vi "ATCcont.vi"() -> ()   [LabVIEW 2014]
doc: "ATC app"
panel:
  in  "정지":bool
  in  "정보1":bool
  in  "도움말":bool
  in  "?":bool
  in  "?":bool
  in  "탭":T1(tab)
  in  "메모":string="필요한 메모를 할수 있습니다. "
  in  "SID&RadarVector. 2":string="SID&RadarVector. "
  in  "인사말":string="인사말"
  in  "CD관제기관":string="관제기관"
  in  "콜사인":string="콜사인\n콜사인\n콜사인"
  in  "도착공항":string="도착공항"
  in  "SID&RadarVector":string="SID&RadarVector"
  in  "비행고도":string="비행고도"
  in  "인사말2":string="인사말"
  in  "콜사인2":string="콜사인"
  in  "콜사인3":string="콜사인"
  in  "콜사인4":string="콜사인"
  in  "콜사인5":string="콜사인"
  in  "콜사인6":string="콜사인"
  in  "도착공항2":string="도착공항"
  in  "제한고도":string="제한고도"
  in  "비행고도2":string="비행고도"
  in  "D접속주파수":string="접속주파수"
  in  "스콱번호":string="스콱번호"
  in  "도착공항3":string="도착공항"
  in  "SID&RadarVector. 3":string="SID&RadarVector. "
  in  "제한고도2":string="제한고도"
  in  "비행고도3":string="비행고도"
  in  "D접속주파수2":string="접속주파수"
  in  "스콱번호2":string="스쾃번호"
  in  "콜사인7":string="콜사인"
  in  "콜사인8":string="콜사인"
  in  "G관제기관":string="관제기관"
  in  "G접속주파수2":string="접속주파수"
  in  "G관제기관2":string="관제기관"
  in  "G접속주파수":string="접속주파수"
  in  "콜사인9":string="콜사인"
  in  "유도로 2":string="유도로"
  in  "유도로":string="유도로"
  in  "방향 2":string="방향"
  in  "방향":string="방향"
  in  "메모2":string="필요한 메모를 할수 있습니다. "
  in  "T관제기관2":string="관제기관"
  in  "콜사인24":string="콜사인"
  in  "T접속주파수2":string="접속주파수"
  in  "T접속주파수":string="접속주파수"
  in  "T관제기관":string="관제기관"
  in  "콜사인23":string="콜사인"
  in  "활주로9":string="활주로"
  in  "G관제기관4":string="관제기관"
  in  "콜사인22":string="콜사인"
  in  "콜사인21":string="콜사인"
  in  "콜사인20":string="콜사인"
  in  "콜사인19":string="콜사인"
  in  "활주로8":string="활주로"
  in  "활주로7":string="활주로"
  in  "콜사인17":string="콜사인"
  in  "활주로6":string="활주로"
  in  "콜사인18":string="콜사인"
  in  "활주로5":string="활주로"
  in  "콜사인16":string="콜사인"
  in  "활주로4":string="활주로"
  in  "콜사인15":string="콜사인"
  in  "활주로3":string="활주로"
  in  "콜사인14":string="콜사인"
  in  "콜사인13":string="콜사인"
  in  "현재기압2":string="현재기압"
  in  "출발공항":string="출발공항"
  in  "활주로2":string="활주로"
  in  "현재기압":string="현재기압"
  in  "출발공항2":string="출발공항"
  in  "활주로1":string="활주로"
  in  "콜사인12":string="콜사인"
  in  "콜사인11":string="콜사인"
  in  "G관제기관3":string="관제기관"
  in  "인사3":string="인사"
  in  "콜사인34 2":string="콜사인"
  in  "D관제기관2":string="관제기관"
  in  "D관제기관":string="관제기관"
  in  "T관제기관3":string="관제기관"
  in  "메모3":string="필요한 메모를 할수 있습니다. "
  in  "인사4":string="인사"
  in  "콜사인25":string="콜사인"
  in  "활주로10":string="활주로"
  in  "콜사인26":string="콜사인"
  in  "바람방향":string="바람방향"
  in  "풍속":string="풍속"
  in  "콜사인28":string="콜사인"
  in  "활주로13":string="활주로"
  in  "콜사인29":string="콜사인"
  in  "활주로12":string="활주로"
  in  "콜사인30":string="콜사인"
  in  "활주로14":string="활주로"
  in  "콜사인31":string="콜사인"
  in  "활주로15":string="활주로"
  in  "T관제기관4":string="관제기관"
  in  "콜사인32":string="콜사인"
  in  "현재고도":string="현재고도"
  in  "허가고도":string="허가고도"
  in  "콜사인33":string="콜사인"
  in  "접속주파수":string="접속주파수"
  in  "콜사인34":string="콜사인"
  in  "접속주파수2":string="접속주파수"
  in  "순항고도or이니셜고도":string="순항고도or이니셜고도"
  in  "D관제기관5":string="관제기관"
  in  "메모 4":string="필요한 메모를 할수 있습니다. "
  in  "인사5":string="인사"
  in  "D관제기관3":string="관제기관"
  in  "콜사인35":string="콜사인"
  in  "현재고도A":string="현재고도"
  in  "콜사인36":string="콜사인"
  in  "D관제기관4":string="관제기관"
  in  "허가고도4":string="허가고도"
  in  "허가고도5":string="허가고도"
  in  "콜사인37":string="콜사인"
  in  "콜사인38":string="콜사인"
  in  "허가고도6":string="허가고도"
  in  "허가고도7":string="허가고도"
  in  "콜사인39":string="콜사인"
  in  "콜사인40":string="콜사인"
  in  "C관제기관":string="관제기관"
  in  "A접속주파수":string="접속주파수"
  in  "C관제기관2":string="관제기관"
  in  "A접속주파수2":string="접속주파수"
  in  "콜사인41":string="콜사인"
  in  "콜사인38 2":string="콜사인"
  in  "D관제기관6":string="관제기관"
  in  "허가고도6 2":string="허가고도"
  in  "허가고도6 3":string="허가고도"
  in  "콜사인39 2":string="콜사인"
  in  "메모5":string="필요한 메모를 할수 있습니다. "
  in  "인사말 2":string="인사말"
  in  "허가고도 2":string="허가고도"
  in  "지점":string="지점"
  in  "허가고도7 2":string="허가고도"
  in  "콜사인38 3":string="콜사인"
  in  "콜사인39 3":string="콜사인"
  in  "허가고도7 3":string="허가고도"
  in  "지점 2":string="지점"
  in  "메모6":string="필요한 메모를 할수 있습니다. "
  in  "A관제기관3":string="관제기관"
  in  "콜사인46":string="콜사인"
  in  "날시정보":string="날시정보"
  in  "고도":string="고도"
  in  "콜사인47":string="콜사인"
  in  "A관제기관4":string="관제기관"
  in  "L활주로":string="활주로"
  in  "도착공항4":string="도착공항"
  in  "현재기압":string="현재기압"
  in  "콜사인48":string="콜사인"
  in  "A관제기관5":string="관제기관"
  in  "L활주로":string="활주로"
  in  "도착공항5":string="도착공항"
  in  "현재기압":string="현재기압"
  in  "콜사인49":string="콜사인"
  in  "고도":string="고도"
  in  "콜사인50":string="콜사인"
  in  "고도":string="고도"
  in  "콜사인51":string="콜사인"
  in  "고도":string="고도"
  in  "고도":string="고도"
  in  "콜사인52":string="콜사인"
  in  "콜사인53":string="콜사인"
  in  "A관제기관":string="관제기관"
  in  "풍속":string="풍속"
  in  "바람방향":string="바람방향"
  in  "L활주로3":string="활주로"
  in  "콜사인54":string="콜사인"
  in  "L활주로":string="활주로"
  in  "콜사인55":string="콜사인"
  in  "A관제기관2":string="관제기관"
  in  "L활주로":string="활주로"
  in  "ILS":string="주파수(ils)"
  in  "콜사인56":string="콜사인"
  in  "L활주로6":string="활주로"
  in  "ILS2":string="주파수(ils)"
  in  "콜사인57":string="콜사인"
  in  "T관제기관":string="관제기관"
  in  "T접속주파수":string="접속주파수"
  in  "콜사인58":string="콜사인"
  in  "콜사인59":string="콜사인"
  in  "관제기관":string="관제기관"
  in  "T접속주파수":string="접속주파수"
  in  "메모7":string="필요한 메모를 할수 있습니다. "
  in  "바람방향":string="바람방향"
  in  "관제기관":string="관제기관"
  in  "콜사인60":string="콜사인"
  in  "L활주로7":string="활주로"
  in  "콜사인61":string="콜사인"
  in  "풍속":string="풍속"
  in  "콜사인62":string="콜사인"
  in  "L활주로":string="활주로"
  in  "L활주로":string="활주로"
  in  "관제기관":string="관제기관"
  in  "콜사인63":string="콜사인"
  in  "관제기관3":string="관제기관"
  in  "콜사인64":string="콜사인"
  in  "L활주로":string="활주로"
  in  "G관제기관":string="관제기관"
  in  "G접속주파수":string="접속주파수"
  in  "콜사인65":string="콜사인"
  in  "관제기관":string="관제기관"
  in  "G접속주파수":string="접속주파수"
  in  "콜사인70":string="콜사인"
  in  "C활주로3":string="활주로"
  in  "C활주로2":string="활주로"
  in  "관제기관3 2":string="관제기관"
  in  "C활주로":string="활주로"
  in  "콜사인69":string="콜사인"
  in  "관제기관2":string="관제기관"
  in  "메모8":string="필요한 메모를 할수 있습니다. "
  in  "관제기관":string="관제기관"
  in  "콜사인66":string="콜사인"
  in  "콜사인67":string="콜사인"
  in  "게이트번호":string="게이트번호"
  in  "THEN":string="then"
  in  "콜사인68":string="콜사인"
  in  "게이트번호2":string="게이트번호"
  in  "THEN2":string="then"
  in  "콜사인10":string="콜사인"
  in  "관제기관4":string="관제기관"
  in  "콜사인71":string="콜사인"
  in  "콜사인72":string="콜사인"
  # "controller.v3.0"
  # "~"
  # "Good"
  # "Clearance Delivery"
  # "Pilot"
  # "at FL"
  # "Request IFR Clearance to"
  # "Airport via"
  # "~"
  # "Good"
  # "Controller"
  # ",  Clearance  Delivery, standby."
  # "Pilot"
  # "Stand by,"
  # "Controller"
  # "Delivery 또는 Delivery, Are you ready to copy?"
  # "Pilot"
  # "Go Ahead 또는 Ready to copy"
  # "Airport via"
  # ", Cleared to"
  # "Controller"
  # "ft expect FL"
  # "then as filed. Climb and Maintain"
  # "Departure Frequency"
  # "Read back."
  # "Squawk"
  # "Pilot"
  # "Airport via"
  # "Cleared to"
  # ","
  # "then as filed."
  # "Climb and Maintain"
  # "ft expect FL"
  # "Departure Frequency"
  # "and  Squawk"
  # "Controller"
  # ", Read back is corrent contact"
  # "Ground"
  # "bye bye~."
  # "Pilot"
  # "Roger, contact"
  # ", bye bye~"
  # "Pilot"
  # "Good"
  # "~"
  # "ready for push back and Engine Start."
  # ","
  # ", Rwy"
  # "Push Back and Engine Start Approved, heading to"
  # "Controller"
  # ","
  # "QNH"
  # "Read Back."
  # "Pilot"
  # "Roger\nPush Back and Engine Start Approved, heading to"
  # ", Rwy"
  # "QNH"
  # "Ready for taxi to the Rwy"
  # ","
  # "Pilot"
  # "- Push back 완료 후 -"
  # ", Ready for Taxi to Rwy"
  # "Controller"
  # ", taxi to"
  # "via taxiway"
  # ", Roger"
  # "Pilot"
  # "via taxiway"
  # "Taxi to"
  # "- 활주로를 건널 상황일 때 -"
  # "Pilot"
  # "Request Cross Rwy"
  # "Controller"
  # ", cleared Cross Rwy"
  # "Pilot"
  # "cleared Cross Rwy"
  # "Controller"
  # "Squawk Mode C."
  # "Pilot"
  # ", Roger squawk mode 'C'"
  # "------------------------ 홀딩 포인트 도착 후 ----------------------------------"
  # "Pilot"
  # "hold short of Rwy"
  # ","
  # "Controller"
  # "Roger,"
  # "contact"
  # "Tower"
  # "bye bye~"
  # "Pilot"
  # "Contact"
  # "Pilot"
  # "Good"
  # "~"
  # ",  hold short Rwy"
  # ", Ready for Departure"
  # "(곧바로 이륙허가)"
  # "Controller"
  # ", wind"
  # "knot, cleared for take off."
  # "at"
  # "(활주로 정렬대기)"
  # "Controller"
  # "Line up and wait Rwy"
  # "Pilot"
  # "Line up and wait Rwy"
  # "Roger,"
  # "(홀딩 포인트에서 대기)"
  # "Controller"
  # ", Hold short rwy"
  # ","
  # "Pilot"
  # "Hold short of Rwy"
  # "Roger,"
  # "- 이 륙 후 -"
  # "Pilot"
  # "ft."
  # "Airborn Passing"
  # "ft, Climbing"
  # ","
  # "Controller"
  # ", contact"
  # "Departure,"
  # "bye bye~"
  # "Pilot"
  # ", Roger"
  # "Contact"
  # "Departure,"
  # "bye bye~"
  # "Good"
  # "~"
  # "Pilot"
  # "Passing"
  # "expect"
  # "with (SID)."
  # ","
  # ","
  # "Controller"
  # "Departure, Radar Contact, Climb via (SID) to"
  # ","
  # "."
  # "Pilot"
  # "Roger, Climb via"
  # ","
  # "-고도제한 해제시-"
  # "Controller"
  # "Departure, Radar Contact, Climb via (SID) to"
  # ", Cancel Level Restrictions."
  # "Pilot"
  # "Roger, Climb via (SID) to"
  # ", Cancel Level Restrictions,"
  # "-속도제한 해제시-"
  # "Controller"
  # "Departure, Radar Contact, Climb via (SID) to"
  # ", Cancel Speed Restrictions."
  # "Pilot"
  # "Roger, Climb via (SID) to"
  # ", Cancel Speed Restrictions,"
  # "Controller"
  # "Control,"
  # ", bye bye."
  # ", You are leaving my airspace, Contact"
  # "Pilot"
  # "Contact"
  # "G'day"
  # "Control,"
  # ","
  # "Pilot"
  # "Good"
  # "Decend and maintain FL"
  # "with (SID)."
  # "-하강 발부-"
  # "Controller"
  # "by"
  # ", Descend and Maintain"
  # "Pilot"
  # "Descend and Maintain"
  # "by"
  # "Pilot"
  # ","
  # "FL"
  # "with information"
  # ","
  # ", Expect vector to ILS Rwy"
  # "approach"
  # "Controller"
  # "QNH"
  # "Roger,"
  # "Pilot"
  # ", Expect vector to ILS Rwy"
  # "final approach"
  # "QNH"
  # "Controller"
  # ", Decend and maintain FL"
  # "Pilot"
  # "Decend and maintain FL"
  # "Roger,"
  # "Controller"
  # ", Decend and maintain"
  # "ft"
  # "Pilot"
  # "Roger"
  # "Decend and maintain"
  # "ft"
  # "Controller"
  # ","
  # "for landing"
  # "wind"
  # "knots active Rwy"
  # "at"
  # "Pilot"
  # "Roger,"
  # "Rwy"
  # "for landing"
  # "Controller"
  # ","
  # "approach use Rwy"
  # "ILS"
  # "Roger,"
  # "Pilot"
  # "Use Rwy"
  # "ILS"
  # "- 정 렬 후 -"
  # "Pilot"
  # "Approach,"
  # ", Established on Localizer."
  # "Controller"
  # "Tower,"
  # "Good day,"
  # "Roger, Contact"
  # "Pilot"
  # "Contact"
  # "Tower"
  # "Good day,"
  # "Pilot"
  # ","
  # "Inbound Approaching Rwy"
  # "Controller"
  # ", Wind"
  # "at"
  # "knots Rwy"
  # ", Cleared to land"
  # "Pilot"
  # "Rwy"
  # "Cleared to land"
  # "Pilot"
  # ","
  # "- 착 륙 후 -"
  # ","
  # "Pilot"
  # "Touch down with Rwy"
  # "Controller"
  # "Roger, change squawk mode Standby and contact"
  # "bye bye~"
  # "ground"
  # "Pilot"
  # ", Roger"
  # "bye bye~"
  # "Change squawk mode standby and contact"
  # "- 활주로를 건널 상황일 때 -"
  # "Pilot"
  # ","
  # "Request Cross Rwy"
  # "Controller"
  # ", Cross Rwy"
  # "approved."
  # "Pilot"
  # "Cross Rwy"
  # "approved"
  # ","
  # "Pilot"
  # "Ready to taxi to the Gate"
  # "Controller"
  # ", taxi to the gate"
  # "via taxi way"
  # "Roger,"
  # "Pilot"
  # "taxi to the gate"
  # "via taxi way"
  # "- 게이트 도착 후 -"
  # "Pilot"
  # "at Gate and Engine Shut down."
  # "Thank you for your ATC service."
  # "Controller"
  # ", at the gate and Engine Shut down, Thank you ~~"
  # "Pilot"
  # "Have a nice day,"
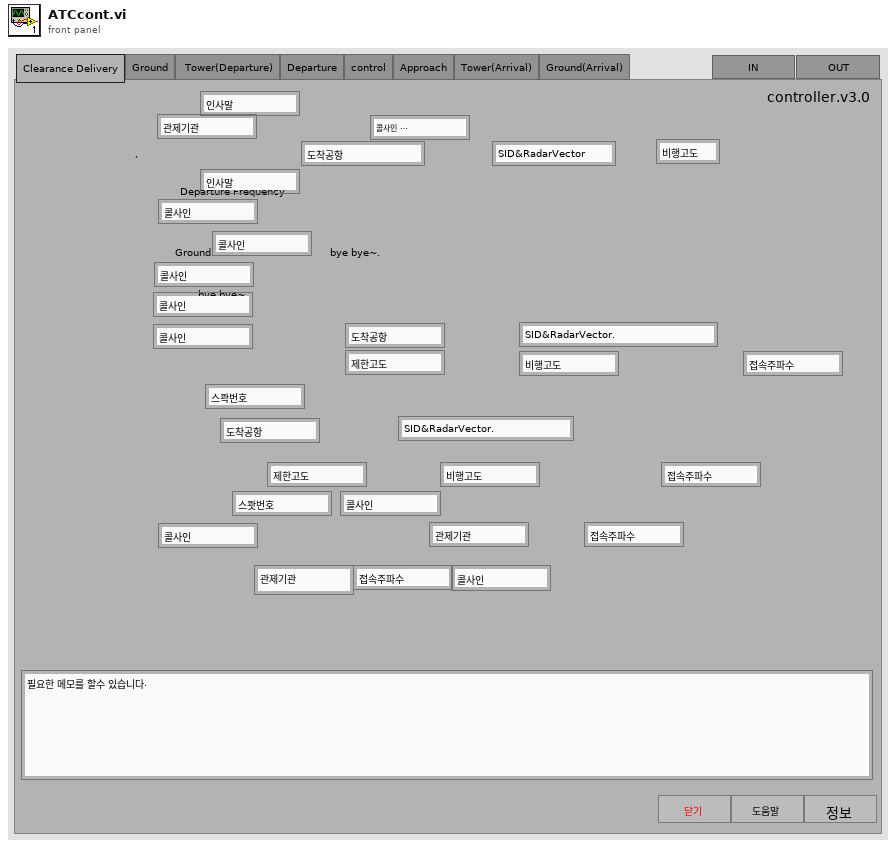
[diagram p1: front panel]
types:
  T1 = enum32{"Clearance Delivery", "Ground", " Tower(Departure)", "Departure", "control", "Approach", "Tower(Arrival)", "Ground(Arrival)"}
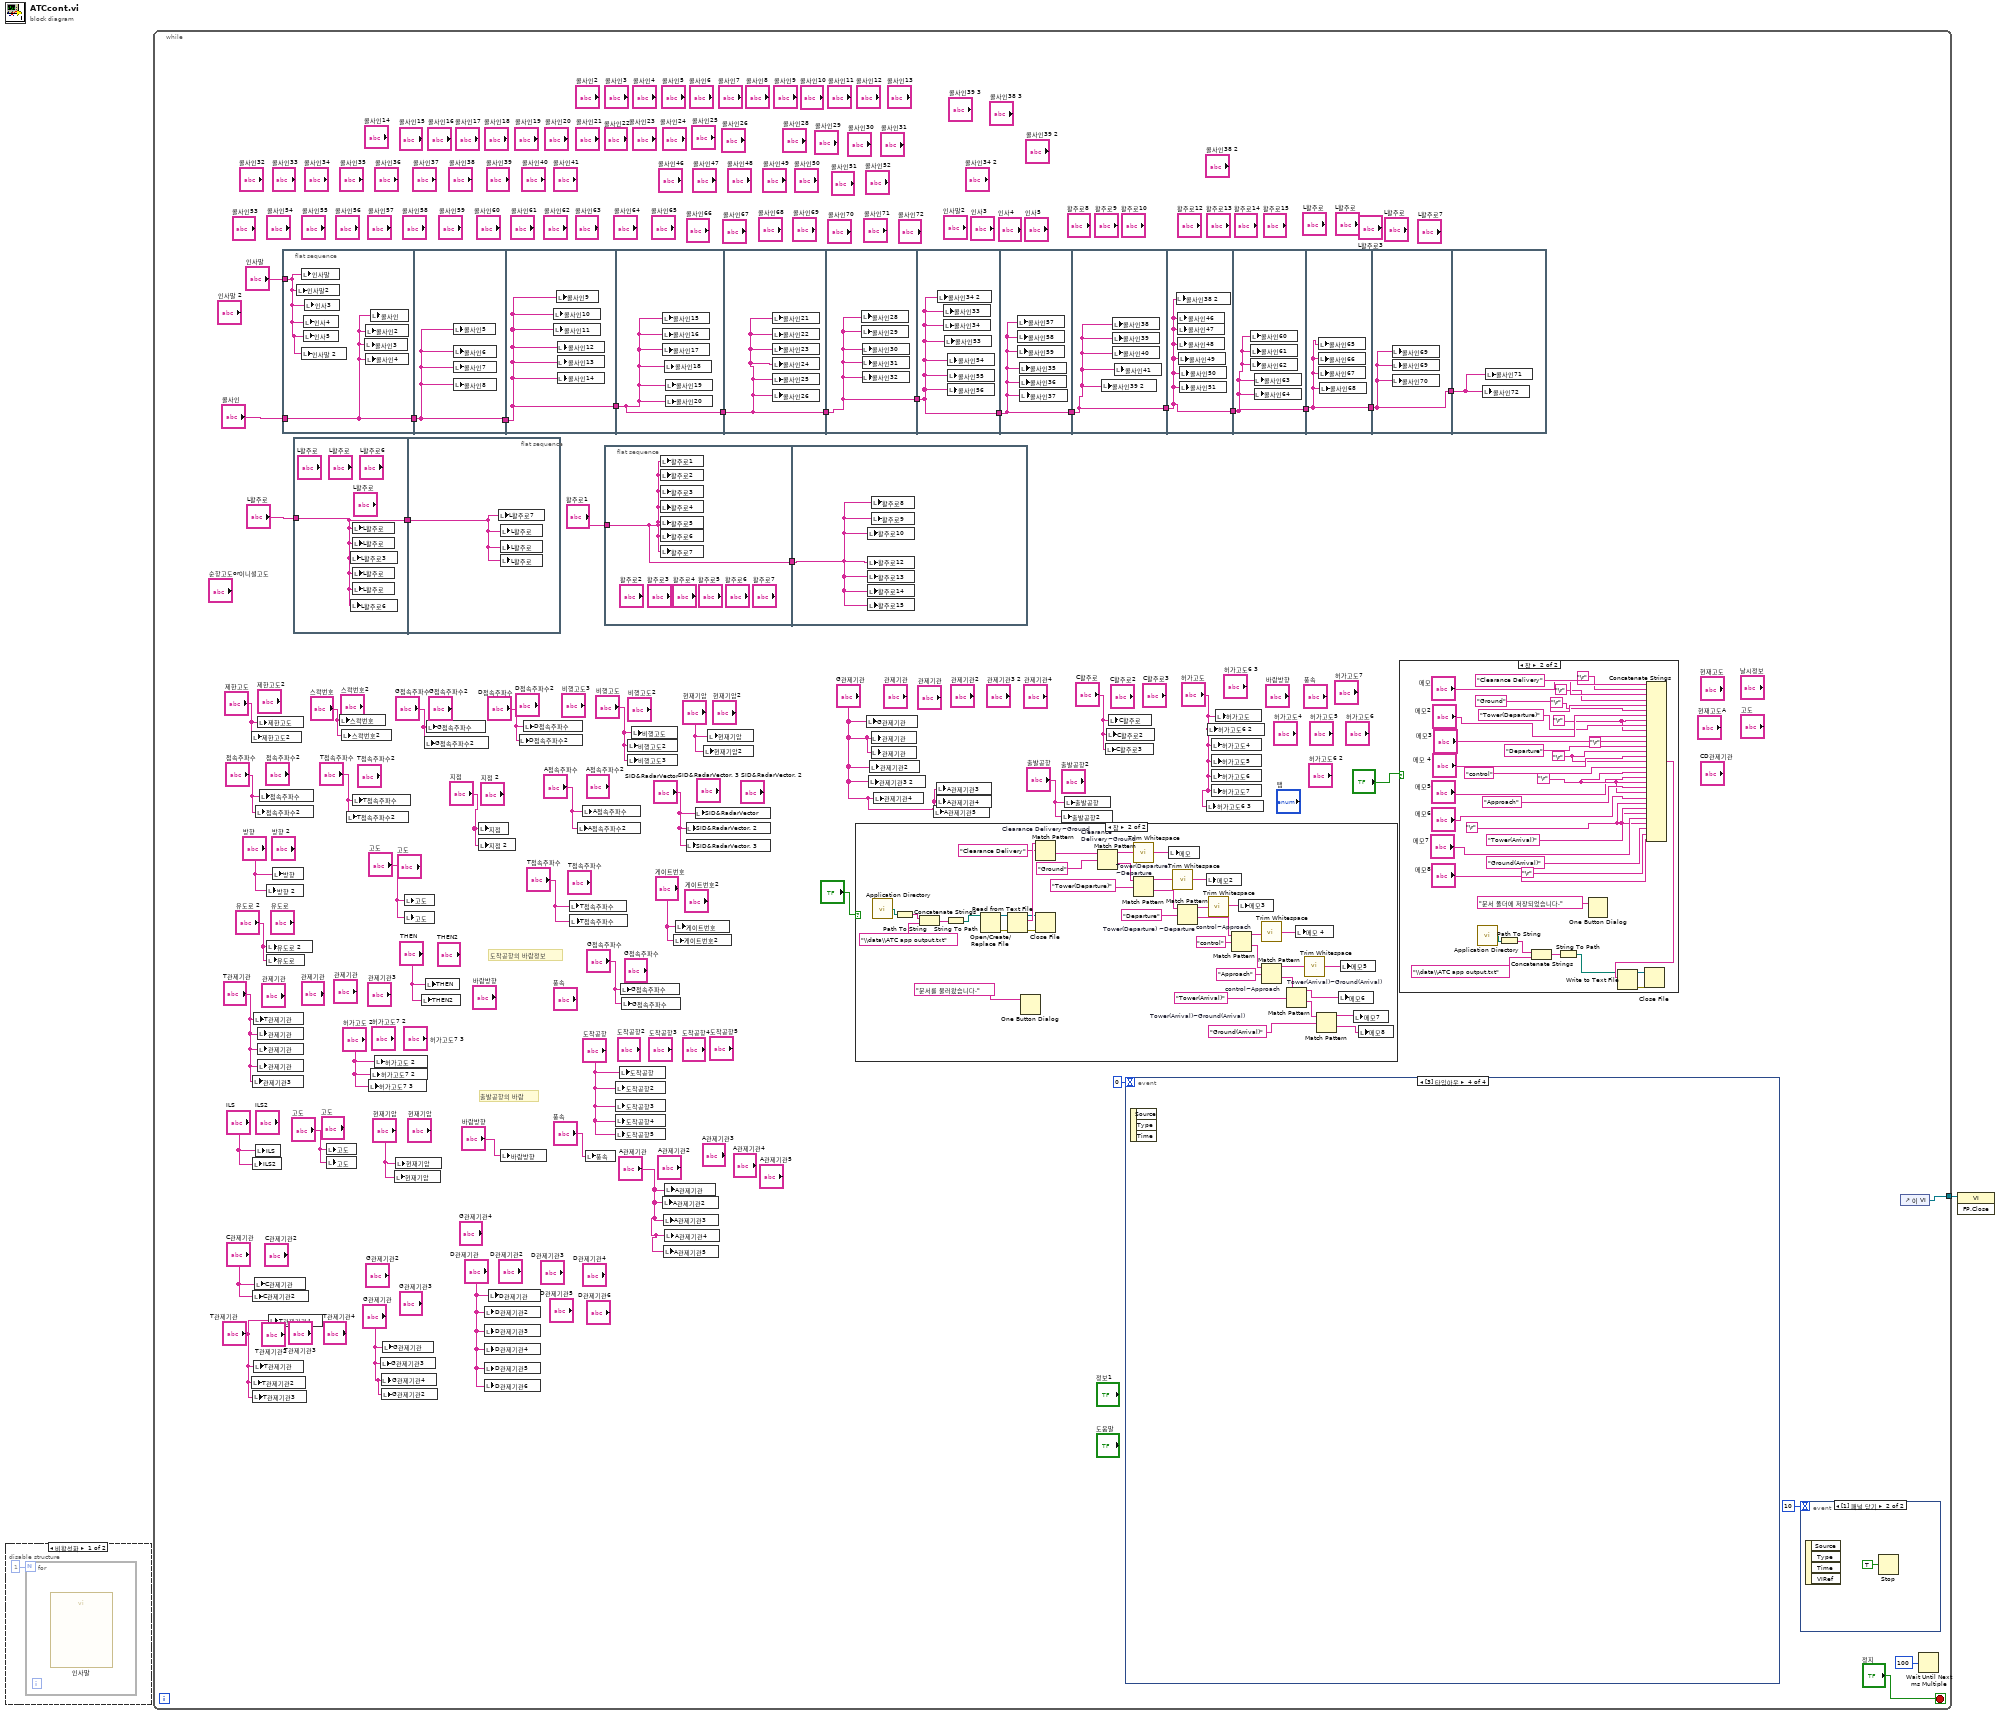
[diagram p0: block diagram]
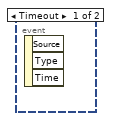
[diagram p2: hidden frame]
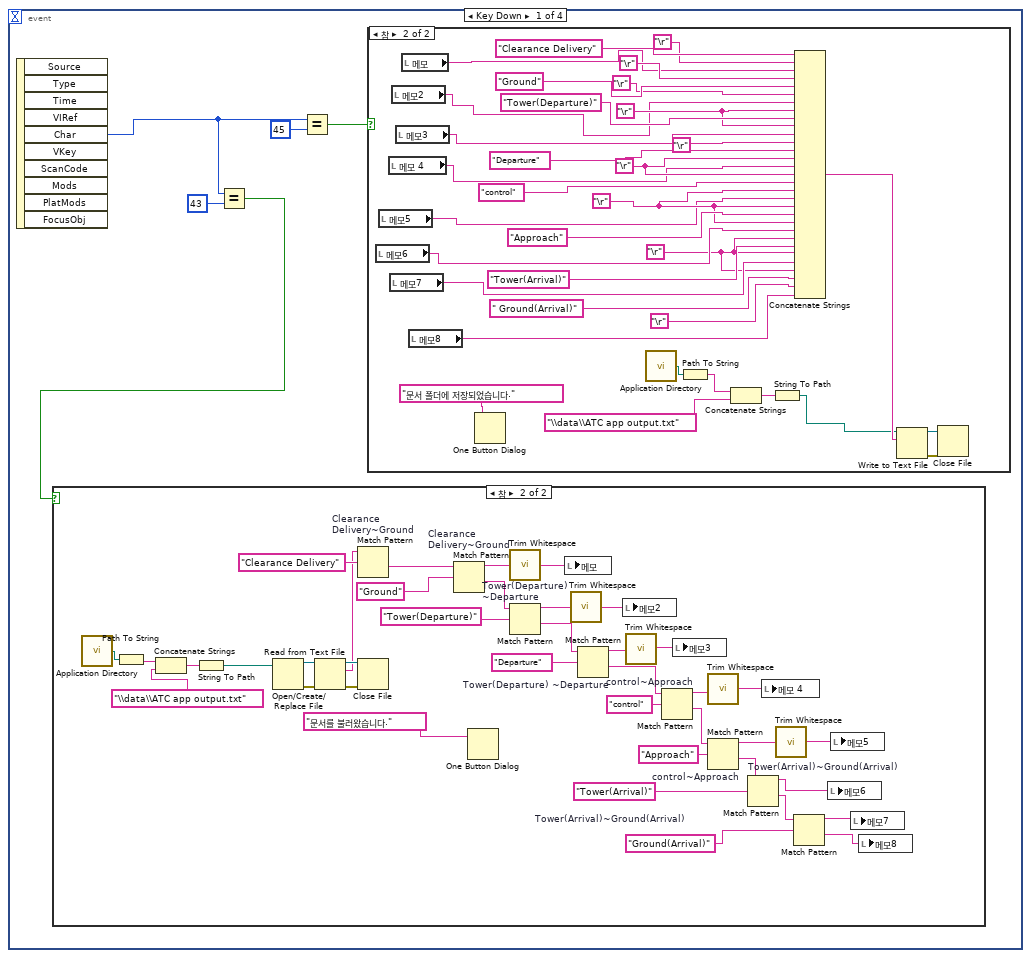
[diagram p3: hidden frame]
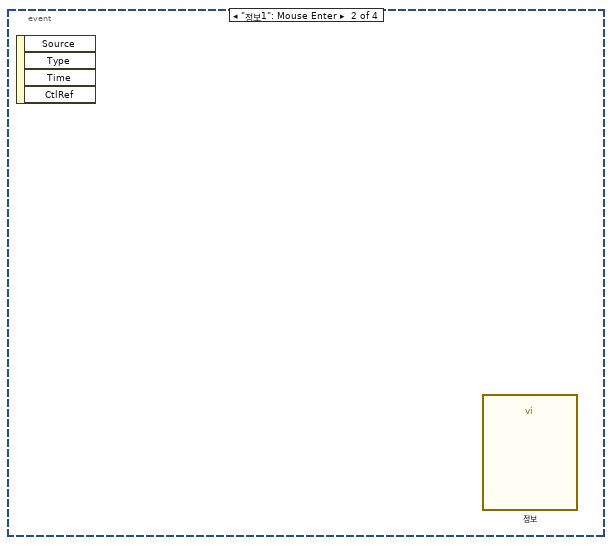
[diagram p6: hidden frame]
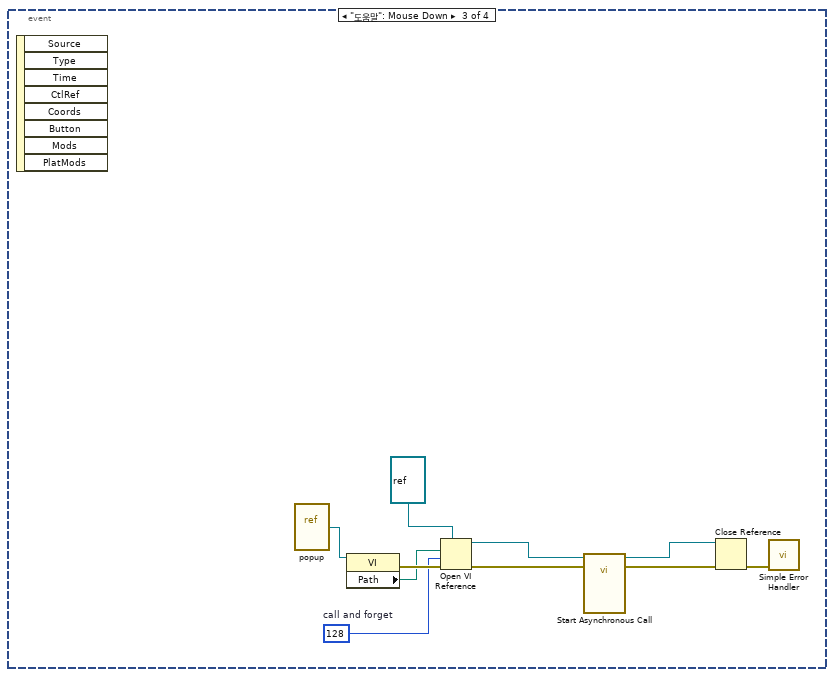
[diagram p7: hidden frame]
diagram:
  n1 = disable-structure shown="비활성화" {
    frame Disabled {
      n2 = for {
        N: 1 -> [_]
        n3 = call "인사말"() -> ()  [unwired: 10 in, 2 out]
      }
    }
    frame Enabled {
    }
  }
  n4 = while {
    tunnel: [w5] -> w1
    stop <- "정지" stop-if-true
    # "출발공항의 바람"
    # "도착공항의 바람정보"
    n5 = local write "제한고도2"("제한고도") -> ()
    n6 = local write "T관제기관2"("T관제기관") -> ()
    n7 = local write "ILS2"("ILS") -> ()
    n8 = local write "관제기관3"("T관제기관") -> ()
    n9 = local write "C관제기관2"("C관제기관") -> ()
    n10 = local write "T관제기관3"("T관제기관") -> ()
    n11 = local write "T관제기관"("T관제기관") -> ()
    n12 = local write "T관제기관"("T관제기관") -> ()
    n13 = local write "C관제기관"("C관제기관") -> ()
    n14 = local write "접속주파수2"("접속주파수") -> ()
    n15 = local write "ILS"("ILS") -> ()
    n16 = local write "제한고도"("제한고도") -> ()
    n17 = local write "관제기관"("T관제기관") -> ()
    n18 = local write "관제기관"("T관제기관") -> ()
    n19 = local write "관제기관"("T관제기관") -> ()
    n20 = local write "접속주파수"("접속주파수") -> ()
    n21 = local write "방향 2"("방향") -> ()
    n22 = local write "유도로 2"("유도로 2") -> ()
    n23 = local write "유도로"("유도로 2") -> ()
    n24 = local write "T관제기관4"("T관제기관") -> ()
    n25 = local write "방향"("방향") -> ()
    n26 = flat-sequence {
      tunnel: [w227] -> w61
      tunnel: "콜사인" -> [w227]
      tunnel: "인사말" -> [w226]
      tunnel: w61 -> [w228]
      tunnel: [w228] -> w60
      tunnel: w60 -> [w229]
      tunnel: [w229] -> w59
      tunnel: w59 -> [w230]
      tunnel: [w230] -> w58
      tunnel: [w231] -> w57
      tunnel: w58 -> [w231]
      tunnel: w57 -> [w232]
      tunnel: [w232] -> w56
      tunnel: [w233] -> w55
      tunnel: w56 -> [w233]
      tunnel: w55 -> [w234]
      tunnel: [w234] -> w54
      tunnel: w54 -> [w235]
      tunnel: [w235] -> w53
      tunnel: w53 -> [w236]
      tunnel: [w236] -> w52
      tunnel: w52 -> [w237]
      tunnel: [w237] -> w51
      tunnel: w51 -> [w238]
      tunnel: [w238] -> w50
      tunnel: w50 -> [w239]
      tunnel: [w239] -> w49
      tunnel: w49 -> [w240]
      frame #0 {
        n27 = local write "인사말2"(w226) -> ()
        n28 = local write "인사말"(w226) -> ()
        n29 = local write "인사말 2"(w226) -> ()
        n30 = local write "인사4"(w226) -> ()
        n31 = local write "인사5"(w226) -> ()
        n32 = local write "인사3"(w226) -> ()
        n33 = local write "콜사인3"(w227) -> ()
        n34 = local write "콜사인2"(w227) -> ()
        n35 = local write "콜사인4"(w227) -> ()
        n36 = local write "콜사인"(w227) -> ()
      }
      frame #1 {
        n37 = local write "콜사인5"(w228) -> ()
        n38 = local write "콜사인6"(w228) -> ()
        n39 = local write "콜사인7"(w228) -> ()
        n40 = local write "콜사인8"(w228) -> ()
      }
      frame #2 {
        n41 = local write "콜사인10"(w229) -> ()
        n42 = local write "콜사인11"(w229) -> ()
        n43 = local write "콜사인9"(w229) -> ()
        n44 = local write "콜사인12"(w229) -> ()
        n45 = local write "콜사인13"(w229) -> ()
        n46 = local write "콜사인14"(w229) -> ()
      }
      frame #3 {
        n47 = local write "콜사인15"(w230) -> ()
        n48 = local write "콜사인16"(w230) -> ()
        n49 = local write "콜사인17"(w230) -> ()
        n50 = local write "콜사인18"(w230) -> ()
        n51 = local write "콜사인19"(w230) -> ()
        n52 = local write "콜사인20"(w230) -> ()
      }
      frame #4 {
        n53 = local write "콜사인21"(w231) -> ()
        n54 = local write "콜사인22"(w231) -> ()
        n55 = local write "콜사인23"(w231) -> ()
        n56 = local write "콜사인24"(w231) -> ()
        n57 = local write "콜사인25"(w231) -> ()
        n58 = local write "콜사인26"(w231) -> ()
      }
      frame #5 {
        n59 = local write "콜사인28"(w232) -> ()
        n60 = local write "콜사인29"(w232) -> ()
        n61 = local write "콜사인30"(w232) -> ()
        n62 = local write "콜사인31"(w232) -> ()
        n63 = local write "콜사인32"(w232) -> ()
      }
      frame #6 {
        n64 = local write "콜사인34 2"(w233) -> ()
        n65 = local write "콜사인33"(w233) -> ()
        n66 = local write "콜사인34"(w233) -> ()
        n67 = local write "콜사인53"(w233) -> ()
        n68 = local write "콜사인54"(w233) -> ()
        n69 = local write "콜사인55"(w233) -> ()
        n70 = local write "콜사인56"(w233) -> ()
      }
      frame #7 {
        n71 = local write "콜사인57"(w234) -> ()
        n72 = local write "콜사인58"(w234) -> ()
        n73 = local write "콜사인59"(w234) -> ()
        n74 = local write "콜사인35"(w234) -> ()
        n75 = local write "콜사인36"(w234) -> ()
        n76 = local write "콜사인37"(w234) -> ()
      }
      frame #8 {
        n77 = local write "콜사인39 2"(w235) -> ()
        n78 = local write "콜사인38"(w235) -> ()
        n79 = local write "콜사인39"(w235) -> ()
        n80 = local write "콜사인40"(w235) -> ()
        n81 = local write "콜사인41"(w235) -> ()
      }
      frame #9 {
        n82 = local write "콜사인38 2"(w236) -> ()
        n83 = local write "콜사인46"(w236) -> ()
        n84 = local write "콜사인47"(w236) -> ()
        n85 = local write "콜사인48"(w236) -> ()
        n86 = local write "콜사인49"(w236) -> ()
        n87 = local write "콜사인50"(w236) -> ()
        n88 = local write "콜사인51"(w236) -> ()
      }
      frame #10 {
        n89 = local write "콜사인60"(w237) -> ()
        n90 = local write "콜사인61"(w237) -> ()
        n91 = local write "콜사인62"(w237) -> ()
        n92 = local write "콜사인63"(w237) -> ()
        n93 = local write "콜사인64"(w237) -> ()
      }
      frame #11 {
        n94 = local write "콜사인65"(w238) -> ()
        n95 = local write "콜사인66"(w238) -> ()
        n96 = local write "콜사인67"(w238) -> ()
        n97 = local write "콜사인68"(w238) -> ()
      }
      frame #12 {
        n98 = local write "콜사인69"(w239) -> ()
        n99 = local write "콜사인69"(w239) -> ()
        n100 = local write "콜사인70"(w239) -> ()
      }
      frame #13 {
        n101 = local write "콜사인72"(w240) -> ()
        n102 = local write "콜사인71"(w240) -> ()
      }
    }
    n103 = flat-sequence {
      tunnel: "L활주로" -> [w243]
      tunnel: [w243] -> w63
      tunnel: w63 -> [w244]
      frame #0 {
        n104 = local write "L활주로3"(w243) -> ()
        n105 = local write "L활주로6"(w243) -> ()
        n106 = local write "L활주로"(w243) -> ()
        n107 = local write "L활주로"(w243) -> ()
        n108 = local write "L활주로"(w243) -> ()
        n109 = local write "L활주로"(w243) -> ()
      }
      frame #1 {
        n110 = local write "L활주로7"(w244) -> ()
        n111 = local write "L활주로"(w244) -> ()
        n112 = local write "L활주로"(w244) -> ()
        n113 = local write "L활주로"(w244) -> ()
      }
    }
    n114 = local write "고도"("고도") -> ()
    n115 = local write "고도"("고도") -> ()
    n116 = local write "스콱번호"("스콱번호") -> ()
    n117 = local write "스콱번호2"("스콱번호") -> ()
    n118 = local write "T접속주파수2"("T접속주파수") -> ()
    n119 = local write "T접속주파수"("T접속주파수") -> ()
    n120 = local write "허가고도7 3"("허가고도 2") -> ()
    n121 = local write "허가고도7 2"("허가고도 2") -> ()
    n122 = local write "허가고도 2"("허가고도 2") -> ()
    n123 = local write "G관제기관3"("G관제기관") -> ()
    n124 = local write "G관제기관4"("G관제기관") -> ()
    n125 = local write "G관제기관2"("G관제기관") -> ()
    n126 = local write "G관제기관"("G관제기관") -> ()
    n127 = local write "현재기압"("현재기압") -> ()
    n128 = local write "현재기압"("현재기압") -> ()
    n129 = local write "고도"("고도") -> ()
    n130 = local write "고도"("고도") -> ()
    n131 = local write "THEN2"("THEN") -> ()
    n132 = local write "G접속주파수2"("G접속주파수") -> ()
    n133 = local write "THEN"("THEN") -> ()
    n134 = local write "G접속주파수"("G접속주파수") -> ()
    n135 = local write "지점"("지점") -> ()
    n136 = local write "지점 2"("지점") -> ()
    n137 = local write "D관제기관2"("D관제기관") -> ()
    n138 = local write "D관제기관3"("D관제기관") -> ()
    n139 = local write "D관제기관4"("D관제기관") -> ()
    n140 = local write "D관제기관5"("D관제기관") -> ()
    n141 = local write "D관제기관6"("D관제기관") -> ()
    n142 = local write "D관제기관"("D관제기관") -> ()
    n143 = local write "바람방향"("바람방향") -> ()
    n144 = local write "D접속주파수2"("D접속주파수") -> ()
    n145 = local write "D접속주파수"("D접속주파수") -> ()
    n146 = local write "T접속주파수"("T접속주파수") -> ()
    n147 = local write "T접속주파수"("T접속주파수") -> ()
    n148 = local write "A접속주파수2"("A접속주파수") -> ()
    n149 = local write "A접속주파수"("A접속주파수") -> ()
    n150 = local write "풍속"("풍속") -> ()
    n151 = flat-sequence {
      tunnel: [w241] -> w62
      tunnel: "활주로1" -> [w241]
      tunnel: w62 -> [w242]
      frame #0 {
        n152 = local write "활주로1"(w241) -> ()
        n153 = local write "활주로2"(w241) -> ()
        n154 = local write "활주로3"(w241) -> ()
        n155 = local write "활주로4"(w241) -> ()
        n156 = local write "활주로5"(w241) -> ()
        n157 = local write "활주로6"(w241) -> ()
        n158 = local write "활주로7"(w241) -> ()
      }
      frame #1 {
        n159 = local write "활주로10"(w242) -> ()
        n160 = local write "활주로12"(w242) -> ()
        n161 = local write "활주로13"(w242) -> ()
        n162 = local write "활주로14"(w242) -> ()
        n163 = local write "활주로15"(w242) -> ()
        n164 = local write "활주로8"(w242) -> ()
        n165 = local write "활주로9"(w242) -> ()
      }
    }
    n166 = local write "도착공항2"("도착공항") -> ()
    n167 = local write "도착공항3"("도착공항") -> ()
    n168 = local write "도착공항4"("도착공항") -> ()
    n169 = local write "도착공항5"("도착공항") -> ()
    n170 = local write "도착공항"("도착공항") -> ()
    n171 = local write "G접속주파수"("G접속주파수") -> ()
    n172 = local write "G접속주파수"("G접속주파수") -> ()
    n173 = local write "비행고도2"("비행고도") -> ()
    n174 = local write "비행고도3"("비행고도") -> ()
    n175 = local write "비행고도"("비행고도") -> ()
    n176 = local write "A관제기관2"("A관제기관") -> ()
    n177 = local write "A관제기관3"("A관제기관") -> ()
    n178 = local write "A관제기관5"("A관제기관") -> ()
    n179 = local write "A관제기관4"("A관제기관") -> ()
    n180 = local write "A관제기관"("A관제기관") -> ()
    n181 = local write "게이트번호2"("게이트번호") -> ()
    n182 = local write "게이트번호"("게이트번호") -> ()
    n183 = local write "SID&RadarVector. 2"("SID&RadarVector") -> ()
    n184 = local write "SID&RadarVector. 3"("SID&RadarVector") -> ()
    n185 = local write "SID&RadarVector"("SID&RadarVector") -> ()
    n186 = local write "현재기압2"("현재기압") -> ()
    n187 = local write "현재기압"("현재기압") -> ()
    n188 = case shown="참" "?" {
      frame False {
      }
      frame True {
        n189 = call <vilib>:"Application Directory.vi"() -> ("Application Directory"=w157:path)
        n190 = Path To String(path=w157) -> (string=w155:string)
        n191 = Concatenate Strings(w155, "\\data\\ATC app output.txt" ("문자열")) -> (w154:string)
        n192 = String To Path(string=w154) -> (path=w153:path)
        n193 = Open/Create/Replace File(file path (use dialog)=w153) -> (refnum out=w171:refnum<file>, error out=w172:errorcluster)  [unwired: 5 in, 1 out]
        n194 = Read from Text File(file (use dialog)=w171, error in=w172) -> (refnum out=w173:refnum<file>, text=w179:string, error out=w174:errorcluster)  [unwired: 2 in, 1 out]
        n195 = One Button Dialog(message="문서를 불러왔습니다." ("메시지")) -> ()  [unwired: 1 in, 1 out]
        n196 = Match Pattern "Clearance Delivery~Ground"(string=w179, regular expression="Clearance Delivery" ("정규식")) -> (after substring=w176:string)  [unwired: 1 in, 3 out]
        n197 = Close File(refnum=w173, error in=w174) -> ()  [unwired: 2 out]
        n198 = Match Pattern "Clearance Delivery~Ground"(string=w176, regular expression="Ground" ("정규식")) -> (before substring=w181:string, after substring=w180:string)  [unwired: 1 in, 2 out]
        n199 = call <vilib>:"Trim Whitespace.vi"("string"=w181) -> ("trimmed string"=w170:string)  [unwired: 1 in]
        n200 = Match Pattern "Tower(Departure) ~Departure"(string=w180, regular expression="Tower(Departure)" ("정규식")) -> (before substring=w182:string, after substring=w185:string)  [unwired: 1 in, 2 out]
        n201 = local write "메모"(w170) -> ()
        n202 = call <vilib>:"Trim Whitespace.vi"("string"=w182) -> ("trimmed string"=w169:string)  [unwired: 1 in]
        n203 = Match Pattern "Tower(Departure) ~Departure"(string=w185, regular expression="Departure" ("정규식")) -> (before substring=w184:string, after substring=w191:string)  [unwired: 1 in, 2 out]
        n204 = local write "메모2"(w169) -> ()
        n205 = call <vilib>:"Trim Whitespace.vi"("string"=w184) -> ("trimmed string"=w168:string)  [unwired: 1 in]
        n206 = Match Pattern "control~Approach"(string=w191, regular expression="control" ("정규식")) -> (before substring=w189:string, after substring=w187:string)  [unwired: 1 in, 2 out]
        n207 = local write "메모3"(w168) -> ()
        n208 = call <vilib>:"Trim Whitespace.vi"("string"=w189) -> ("trimmed string"=w167:string)  [unwired: 1 in]
        n209 = Match Pattern "control~Approach"(string=w187, regular expression="Approach" ("정규식")) -> (before substring=w190:string, after substring=w164:string)  [unwired: 1 in, 2 out]
        n210 = Match Pattern "Tower(Arrival)~Ground(Arrival)"(string=w164, regular expression="Tower(Arrival)" ("정규식")) -> (before substring=w162:string, after substring=w160:string)  [unwired: 1 in, 2 out]
        n211 = local write "메모 4"(w167) -> ()
        n212 = call <vilib>:"Trim Whitespace.vi"("string"=w190) -> ("trimmed string"=w166:string)  [unwired: 1 in]
        n213 = Match Pattern "Tower(Arrival)~Ground(Arrival)"(string=w160, regular expression="Ground(Arrival)" ("정규식")) -> (before substring=w159:string, after substring=w158:string)  [unwired: 1 in, 2 out]
        n214 = local write "메모6"(w162) -> ()
        n215 = local write "메모5"(w166) -> ()
        n216 = local write "메모7"(w159) -> ()
        n217 = local write "메모8"(w158) -> ()
      }
    }
    n218 = local write "G관제기관"("G관제기관") -> ()
    n219 = local write "관제기관3 2"("G관제기관") -> ()
    n220 = local write "관제기관2"("G관제기관") -> ()
    n221 = local write "관제기관"("G관제기관") -> ()
    n222 = local write "관제기관"("G관제기관") -> ()
    n223 = local write "관제기관4"("G관제기관") -> ()
    n224 = local write "A관제기관5"("G관제기관") -> ()
    n225 = local write "A관제기관3"("G관제기관") -> ()
    n226 = local write "A관제기관4"("G관제기관") -> ()
    n227 = local write "출발공항2"("출발공항") -> ()
    n228 = local write "출발공항"("출발공항") -> ()
    n229 = local write "C활주로3"("C활주로") -> ()
    n230 = local write "C활주로2"("C활주로") -> ()
    n231 = local write "C활주로"("C활주로") -> ()
    n232 = event shown="[3] 타임아웃" {
      selector: _ -> [_ _ _ _]
      dyn-events: _ -> [_ _ _ _]
      timeout: 0 -> [_ _ _ _]
      event Key Down {
        n233 = event-data() -> ("Char"=w66:i16)  [unwired: 1 in, 9 out]
        n234 = Equal?(x=w66, y=i16 43) -> (x = y?=w67:bool)
        n235 = case shown="참" w67 {
          frame False {
          }
          frame True {
            n236 = call <vilib>:"Application Directory.vi"() -> ("Application Directory"=w74:path)
            n237 = Path To String(path=w74) -> (string=w72:string)
            n238 = Concatenate Strings(w72, "\\data\\ATC app output.txt" ("문자열")) -> (w71:string)
            n239 = String To Path(string=w71) -> (path=w70:path)
            n240 = Open/Create/Replace File(file path (use dialog)=w70) -> (refnum out=w95:refnum<file>, error out=w94:errorcluster)  [unwired: 5 in, 1 out]
            n241 = Read from Text File(file (use dialog)=w95, error in=w94) -> (refnum out=w93:refnum<file>, text=w87:string, error out=w92:errorcluster)  [unwired: 2 in, 1 out]
            n242 = Match Pattern "Clearance Delivery~Ground"(string=w87, regular expression="Clearance Delivery" ("정규식")) -> (after substring=w90:string)  [unwired: 1 in, 3 out]
            n243 = Close File(refnum=w93, error in=w92) -> ()  [unwired: 2 out]
            n244 = Match Pattern "Clearance Delivery~Ground"(string=w90, regular expression="Ground" ("정규식")) -> (before substring=w85:string, after substring=w86:string)  [unwired: 1 in, 2 out]
            n245 = One Button Dialog(message="문서를 불러왔습니다." ("메시지")) -> ()  [unwired: 1 in, 1 out]
            n246 = call <vilib>:"Trim Whitespace.vi"("string"=w85) -> ("trimmed string"=w96:string)  [unwired: 1 in]
            n247 = Match Pattern "Tower(Departure) ~Departure"(string=w86, regular expression="Tower(Departure)" ("정규식")) -> (before substring=w84:string, after substring=w81:string)  [unwired: 1 in, 2 out]
            n248 = local write "메모"(w96) -> ()
            n249 = call <vilib>:"Trim Whitespace.vi"("string"=w84) -> ("trimmed string"=w97:string)  [unwired: 1 in]
            n250 = Match Pattern "Tower(Departure) ~Departure"(string=w81, regular expression="Departure" ("정규식")) -> (before substring=w82:string, after substring=w75:string)  [unwired: 1 in, 2 out]
            n251 = local write "메모2"(w97) -> ()
            n252 = call <vilib>:"Trim Whitespace.vi"("string"=w82) -> ("trimmed string"=w98:string)  [unwired: 1 in]
            n253 = Match Pattern "control~Approach"(string=w75, regular expression="control" ("정규식")) -> (before substring=w77:string, after substring=w79:string)  [unwired: 1 in, 2 out]
            n254 = local write "메모3"(w98) -> ()
            n255 = call <vilib>:"Trim Whitespace.vi"("string"=w77) -> ("trimmed string"=w99:string)  [unwired: 1 in]
            n256 = Match Pattern "control~Approach"(string=w79, regular expression="Approach" ("정규식")) -> (before substring=w76:string, after substring=w102:string)  [unwired: 1 in, 2 out]
            n257 = Match Pattern "Tower(Arrival)~Ground(Arrival)"(string=w102, regular expression="Tower(Arrival)" ("정규식")) -> (before substring=w104:string, after substring=w106:string)  [unwired: 1 in, 2 out]
            n258 = local write "메모 4"(w99) -> ()
            n259 = call <vilib>:"Trim Whitespace.vi"("string"=w76) -> ("trimmed string"=w100:string)  [unwired: 1 in]
            n260 = Match Pattern "Tower(Arrival)~Ground(Arrival)"(string=w106, regular expression="Ground(Arrival)" ("정규식")) -> (before substring=w107:string, after substring=w108:string)  [unwired: 1 in, 2 out]
            n261 = local write "메모6"(w104) -> ()
            n262 = local write "메모5"(w100) -> ()
            n263 = local write "메모7"(w107) -> ()
            n264 = local write "메모8"(w108) -> ()
          }
        }
        n265 = Equal?(x=w66, y=i16 45) -> (x = y?=w69:bool)
        n266 = case shown="참" w69 {
          frame False {
          }
          frame True {
            w117 = "\r"
            w129 = "\r"
            w131 = "\r"
            w134 = "\r"
            n267 = local read "메모6"() -> (w120:string)
            n268 = local read "메모5"() -> (w121:string)
            n269 = local read "메모 4"() -> (w122:string)
            n270 = local read "메모7"() -> (w118:string)
            n271 = local read "메모2"() -> (w124:string)
            n272 = local read "메모3"() -> (w123:string)
            n273 = local read "메모"() -> (w125:string)
            n274 = local read "메모8"() -> (w114:string)
            n275 = One Button Dialog(message="문서 폴더에 저장되었습니다." ("메시지")) -> ()  [unwired: 1 in, 1 out]
            n276 = call <vilib>:"Application Directory.vi"() -> ("Application Directory"=w113:path)
            n277 = Path To String(path=w113) -> (string=w111:string)
            n278 = Concatenate Strings(w111, "\\data\\ATC app output.txt" ("문자열")) -> (w110:string)
            n279 = String To Path(string=w110) -> (path=w109:path)
            n280 = Concatenate Strings("Clearance Delivery", "\r", w125, "\r", "Ground", "\r", w124, w134, "Tower(Departure)", w134, w123, "\r", "Departure", w131, w122, w131, "control", w129, w121, w129, "Approach", w129, w120, w117, "Tower(Arrival)", w117, w118, w117, " Ground(Arrival)", "\r", w114) -> (w128:string)
            n281 = Write to Text File(file (use dialog)=w109, text=w128) -> (refnum out=w142:refnum<file>, error out=w141:errorcluster)  [unwired: 2 in, 1 out]
            n282 = Close File(refnum=w142, error in=w141) -> ()  [unwired: 2 out]
          }
        }
      }
      event "정보1": Mouse Enter {
        n283 = event-data() -> ()  [unwired: 1 in, 4 out]
        n284 = call "정보"() -> ()  [unwired: 10 in, 2 out]
      }
      event "도움말": Mouse Down {
        w143 = 128  # call and forget
        n285 = event-data() -> ()  [unwired: 1 in, 8 out]
        n286 = vi-ref "popup.vi"() -> (w150:refnum<vi>)
        n287 = property class="VI"(reference=w150) -> (error out=w149:errorcluster, "Path"=w148:path)  [unwired: 1 in, 1 out]
        n288 = Open VI Reference(type specifier VI Refnum (for type only)=refnum<vi> refnum, vi path=w148, options=w143, error in (no error)=w149) -> (vi reference=w151:refnum<vi>, error out=w145:errorcluster)  [unwired: 2 in]
        n289 = call-by-ref "Start Asynchronous Call"(reference=w151, error in=w145) -> (reference out=w152:refnum<vi>, error out=w146:errorcluster)  [unwired: 12 in]
        n290 = Close Reference(reference=w152, error in (no error)=w146) -> (error out=w147:errorcluster)
        n291 = call <vilib>:"Simple Error Handler.vi"("error in (no error)"=w147) -> ()  [unwired: 4 in, 5 out]
      }
      event Timeout {
        n292 = event-data() -> ()  [unwired: 1 in, 3 out]
      }
    }
    n293 = local write "허가고도6 3"("허가고도") -> ()
    n294 = local write "허가고도6 2"("허가고도") -> ()
    n295 = local write "허가고도4"("허가고도") -> ()
    n296 = local write "허가고도5"("허가고도") -> ()
    n297 = local write "허가고도6"("허가고도") -> ()
    n298 = local write "허가고도7"("허가고도") -> ()
    n299 = local write "허가고도"("허가고도") -> ()
    n300 = case shown="참" "?" {
      frame False {
      }
      frame True {
        w200 = "\r"
        w207 = "\r"
        w210 = "\r"
        w215 = "\r"
        n301 = call <vilib>:"Application Directory.vi"() -> ("Application Directory"=w196:path)
        n302 = Path To String(path=w196) -> (string=w194:string)
        n303 = Concatenate Strings(w194, "\\data\\ATC app output.txt" ("문자열")) -> (w193:string)
        n304 = String To Path(string=w193) -> (path=w192:path)
        n305 = One Button Dialog(message="문서 폴더에 저장되었습니다." ("메시지")) -> ()  [unwired: 1 in, 1 out]
        n306 = Concatenate Strings("Clearance Delivery", "\r", "메모", "\r", "Ground", "\r", "메모2", w215, "Tower(Departure)", w215, "메모3", "\r", "Departure", w210, "메모 4", w210, "control", w207, "메모5", w207, "Approach", w207, "메모6", w200, "Tower(Arrival)", w200, "메모7", w200, "Ground(Arrival)", "\r", "메모8") -> (w206:string)
        n307 = Write to Text File(file (use dialog)=w192, text=w206) -> (refnum out=w225:refnum<file>, error out=w224:errorcluster)  [unwired: 2 in, 1 out]
        n308 = Close File(refnum=w225, error in=w224) -> ()  [unwired: 2 out]
      }
    }
    n309 = event shown="[1] 패널 닫기" {
      selector: _ -> [_ _]
      dyn-events: _ -> [_ _]
      timeout: 10 -> [_ _]
      event Timeout {
        n310 = event-data() -> ()  [unwired: 1 in, 3 out]
      }
      event Panel Close {
        n311 = event-data() -> ()  [unwired: 1 in, 4 out]
        n312 = Stop(stop? (T)=TRUE ("정지? (참)")) -> ()
      }
    }
    n313 = control-ref of="이 VI"() -> (w5:refnum<vi>)
    n314 = Wait Until Next ms Multiple(millisecond multiple=u32 100 ("ms 배수")) -> ()  [unwired: 1 out]
  }
  n315 = invoke class="VI" method="FP.Close"(reference=w1) -> ()  [unwired: 2 in, 3 out]
